vi "Showing more than one graphs at the same coordinate system.vi"() -> ()   [LabVIEW 2024]
panel:
  out "y=x & y=x^2 Graph":cluster{"Array 3":dbl[], "Array 4":dbl[]}[](graph)
  in  "Array 4":dbl[](array[numeric])
  in  "Array 3":dbl[](array[numeric])
  in  "Array 2":dbl[](array[numeric])
  in  "Array":dbl[](array[numeric])
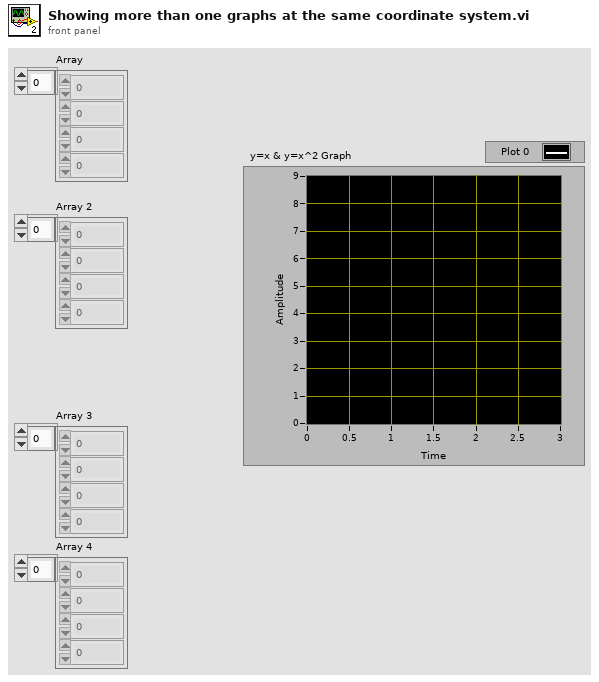
[diagram p1: front panel]
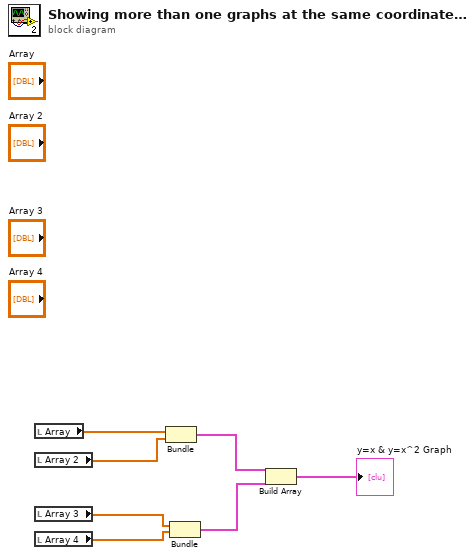
[diagram p0: block diagram]
diagram:
  n1 = local read "Array"() -> (w7:dbl[])
  n2 = local read "Array 2"() -> (w6:dbl[])
  n3 = local read "Array 3"() -> (w5:dbl[])
  n4 = local read "Array 4"() -> (w4:dbl[])
  n5 = Bundle "Bundle"("Array"=w7, "Array 2"=w6) -> (w3:cluster{"Array":dbl[], "Array 2":dbl[]})  [unwired: 1 in]
  n6 = Bundle "Bundle"("Array 3"=w5, "Array 4"=w4) -> (w2:cluster{"Array 3":dbl[], "Array 4":dbl[]})  [unwired: 1 in]
  n7 = Build Array "Build Array"(w3, w2) -> (→"y=x & y=x^2 Graph":cluster{"Array 3":dbl[], "Array 4":dbl[]}[])
